vi "Get Startup Settings.vi"(8 "error in (no error)":errorcluster) -> (0 "error out":errorcluster, 3 "Startup Settings":T1)   [LabVIEW 2023]
doc: "This VI gets the startup seetings for the controller. These same settings can be found and set in NI MAX or with WIF."
uses:
  Type Definitions/Startup Settings.ctl
  Type Definitions/Enum - Metadata.ctl
  Type Definitions/Payload Class.ctl
  <resource>/objmgr/nicriosae.rc
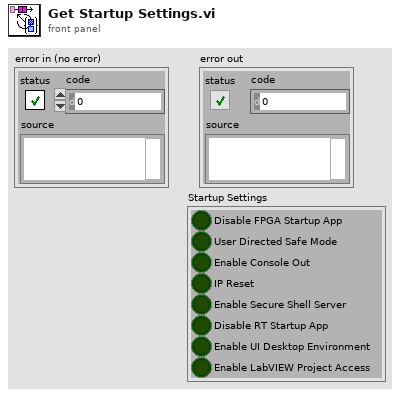
[diagram p1: front panel]
types:
  T1 = typedef "Startup Settings.ctl" = cluster{"Disable FPGA Startup App":bool, "User Directed Safe Mode":bool, "Enable Console Out":bool, "IP Reset":bool, "Enable Secure Shell Server":bool, "Disable RT Startup App":bool, "Enable UI Desktop Environment":bool, "Enable LabVIEW Project Access":bool}
  T2 = typedef "Payload Class.ctl" = enum16{"System State", "Parameters", "Metadata", "Software Monitor", "Data", "Commands"}
  T3 = typedef "Enum - Metadata.ctl" = enum16{"Computer Metadata", "Computer Resources", "RT Image Metadata", "Startup Settings", "Telemetry Recorder Status"}
  T4 = typedef "System Resources.ctl" = cluster{"System Session":refnum<k21>, "System Resource":refnum<k20>, "FPGA VI Reference":refnum<k20>}
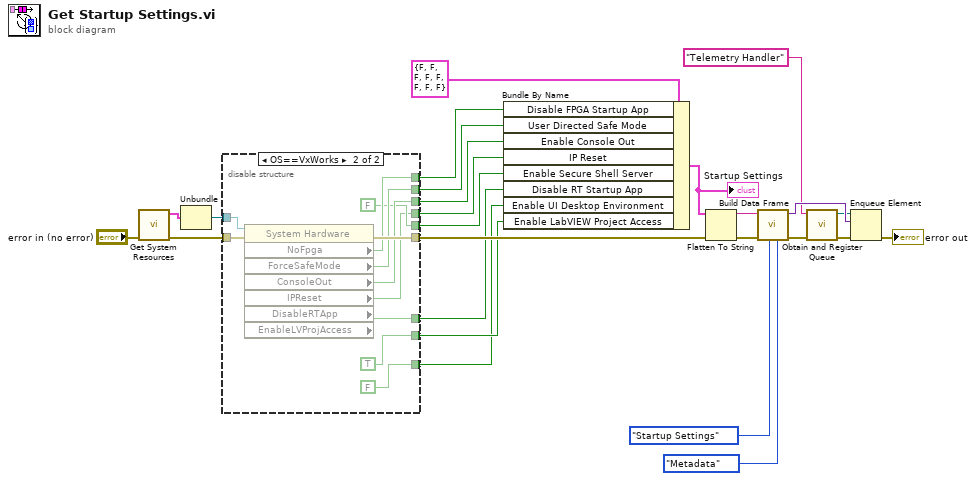
[diagram p0: block diagram]
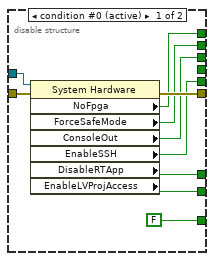
[diagram p2: hidden frame]
diagram:
  n1 = call "Get System Resources.vi"("error in (no error)"="error in (no error)") -> ("error out"=w12:errorcluster, "System Resources"=w4:T4)  [unwired: 9 in]
  n2 = Unbundle(w4) -> ("System Resource"=w11:refnum<k20>)  [unwired: 2 out]
  n3 = disable-structure shown="OS==VxWorks" {
    disable-tunnel: [w35 w46] -> w24
    disable-tunnel: w12 -> [w34 w45]
    disable-tunnel: w11 -> [w33 w44]
    disable-tunnel: [w32 w43] -> w10
    disable-tunnel: [w31 w42] -> w9
    disable-tunnel: [w30 w41] -> w8
    disable-tunnel: [w29 FALSE ("EnableSSH")] -> w7
    disable-tunnel: [w28 w37] -> w1
    disable-tunnel: [w27 TRUE ("EnableLVProjAccess")] -> w6
    disable-tunnel: [FALSE ("Enable UI Desktop Environment") FALSE ("Enable UI Desktop Environment")] -> w3
    disable-tunnel: [_ w36] -> w2
    frame condition #0 (active) {
      n4 = property class="System Hardware"(reference=w33, error in=w34) -> (error out=w35:errorcluster, "NoFpga"=w32:bool, "ForceSafeMode"=w31:bool, "ConsoleOut"=w30:bool, "EnableSSH"=w29:bool, "DisableRTApp"=w28:bool, "EnableLVProjAccess"=w27:bool)  [unwired: 1 out]
    }
    frame condition #1 {
      n5 = property class="System Hardware" props=["NoFpga", "ForceSafeMode", "ConsoleOut", "IPReset", "DisableRTApp", "EnableLVProjAccess"](reference=w44, error in=w45) -> (error out=w46:errorcluster, "NoFpga"=w43:bool, "ForceSafeMode"=w42:bool, "ConsoleOut"=w41:bool, "IPReset"=w36:bool, "DisableRTApp"=w37:bool)  [unwired: 2 out]
    }
  }
  n6 = Bundle By Name(cluster=T1 {"Disable FPGA Startup App"=FALSE, "User Directed Safe Mode"=FALSE, "Enable Console Out"=FALSE, "IP Reset"=FALSE, "Enable Secure Shell Server"=FALSE, "Disable RT Startup App"=FALSE, "Enable UI Desktop Environment"=FALSE, "Enable LabVIEW Project Access"=FALSE}, "Disable FPGA Startup App"=w10, "User Directed Safe Mode"=w9, "Enable Console Out"=w8, "IP Reset"=w2, "Enable Secure Shell Server"=w7, "Disable RT Startup App"=w1, "Enable UI Desktop Environment"=w3, "Enable LabVIEW Project Access"=w6) -> (w23:T1)
  "Startup Settings" <- w23
  n7 = Flatten To String(anything=w23, error in (no error)=w24) -> (data string=w14:string, error out=w17:errorcluster)  [unwired: 2 in, 1 out]
  n8 = call "Build Data Frame.vi"("Payload Class (Data)"=Payload_Class."Metadata", "Payload ID (0)"=Enum_-_Metadata."Startup Settings", "error in (no error)"=w17, "Payload (Empty String)"=w14) -> ("error out"=w21:errorcluster, "Frame"=w20:variant)  [unwired: 6 in]
  n9 = call "Obtain and Register Queue.vi"("error in (no error)"=w21, "Queue Name (unnamed)"="Telemetry Handler" ("name (unnamed)")) -> ("error out"=w22:errorcluster, "Queue Reference"=w19:refnum<queue>)  [unwired: 8 in]
  n10 = Enqueue Element(queue=w19, element=w20, error in (no error)=w22) -> (error out=→"error out":errorcluster)  [unwired: 1 in, 2 out]
